vi "Get Tray.vi"(8 "error in":errorcluster, 9 "Grasp":bool=TRUE, 11 "picture":refnum<vi>) -> (0 "error out":errorcluster, 5 "picture":picture)   [LabVIEW 2013]
uses:
  Arm Globals.vi
  ROS/Code/SubVIs/BaxterSide.ctl
  Prim/Fwd Kenimatics - array.vi
  Move/Move Axis.vi
  <vilib>/Analysis/Matrix/NI_Matrix.lvlib
  <vilib>/Analysis/Matrix/Numeric/Multiply/Multiply - RM,RM.vi
  Move/Move XYA.vi
panel:
  out "Range":dbl
  out "result":cluster{"x":dbl, "y":dbl, "a":dbl}
  # "Y"
  # "X"
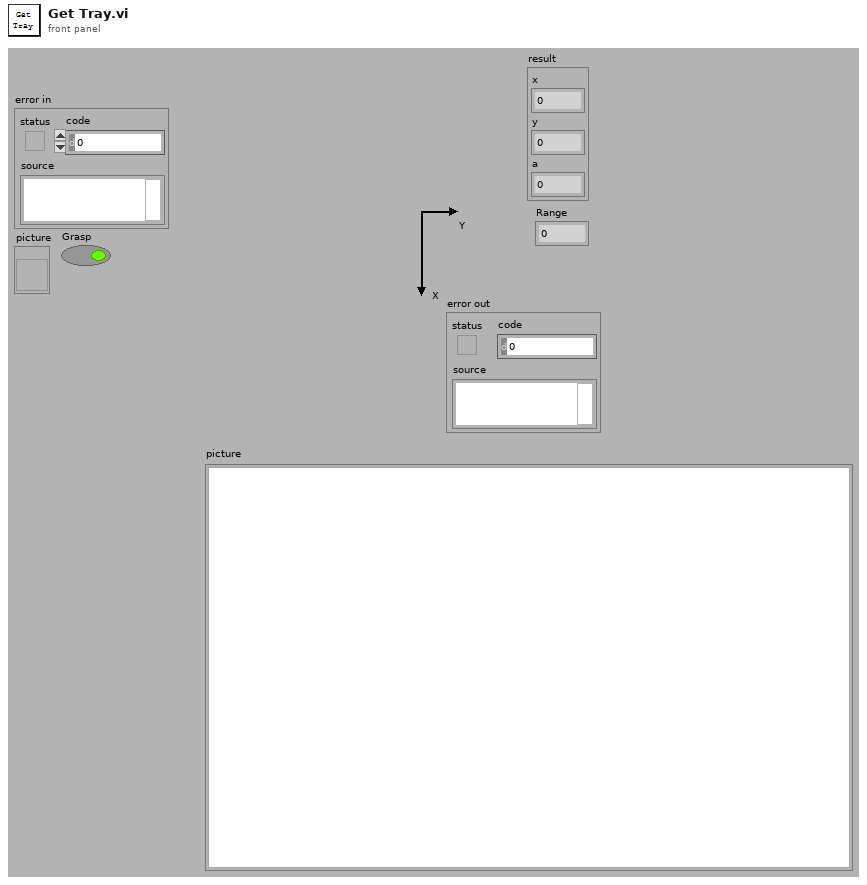
[diagram p1: front panel]
types:
  T1 = typedef "BaxterSide.ctl" = enum16{"left", "right"}
  T2 = typedef "NI_Matrix.lvlib/RealMatrix.ctl" = dbl[][]
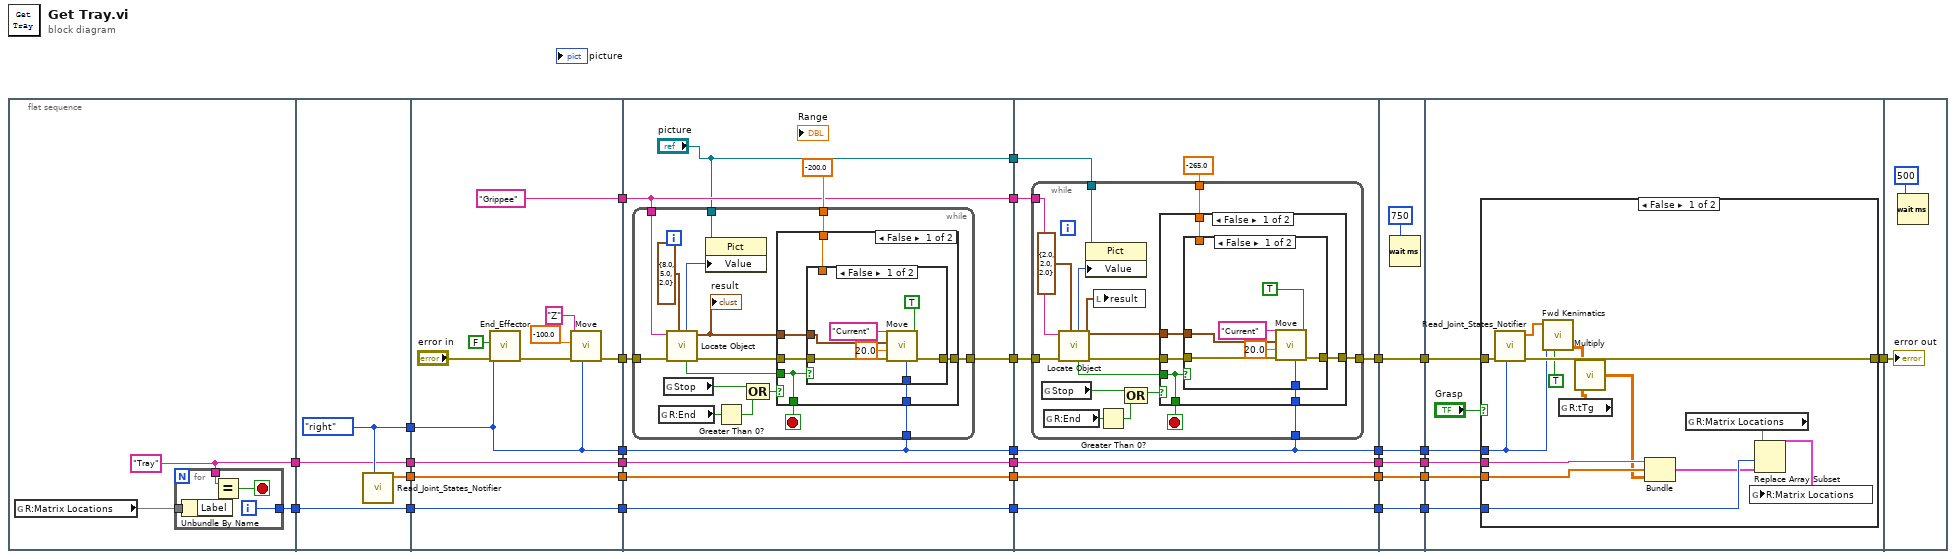
[diagram p0: block diagram]
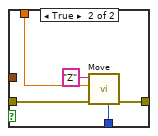
[diagram p2: hidden frame]
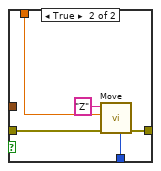
[diagram p4: hidden frame]
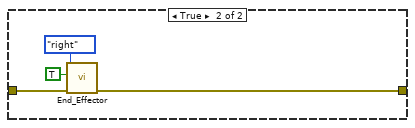
[diagram p6: hidden frame]
diagram:
  n1 = flat-sequence {
    tunnel: [w32] -> w15
    tunnel: [w31] -> w13
    tunnel: [w42] -> w18
    tunnel: [w41] -> w17
    tunnel: [w40] -> w16
    tunnel: w15 -> [w40]
    tunnel: [w39] -> w14
    tunnel: w13 -> [w39]
    tunnel: [w48] -> w30
    tunnel: [w50] -> w29
    tunnel: ["Grippee" ("element")] -> w28
    tunnel: w18 -> [w48]
    tunnel: w17 -> [w46]
    tunnel: w16 -> [w45]
    tunnel: w14 -> [w47]
    tunnel: [w47] -> w12
    tunnel: [w46] -> w11
    tunnel: [w45] -> w10
    tunnel: w30 -> [w59]
    tunnel: w29 -> [w60]
    tunnel: w28 -> [w58]
    tunnel: [w62] -> w27
    tunnel: [w59] -> w26
    tunnel: [w58] -> w25
    tunnel: ["picture"] -> w22
    tunnel: w12 -> [w54]
    tunnel: w11 -> [w55]
    tunnel: w10 -> [w56]
    tunnel: [w56] -> w9
    tunnel: [w55] -> w8
    tunnel: [w54] -> w7
    tunnel: w27 -> [w106]
    tunnel: w26 -> [w102]
    tunnel: w25 -> [w105]
    tunnel: [w104] -> w23
    tunnel: w22 -> [w103]
    tunnel: [w102] -> w20
    tunnel: w9 -> [w101]
    tunnel: w8 -> [w100]
    tunnel: w7 -> [w99]
    tunnel: [w101] -> w5
    tunnel: [w100] -> w3
    tunnel: [w99] -> w1
    tunnel: [w148] -> w24
    tunnel: w23 -> [w148]
    tunnel: [w147] -> w21
    tunnel: w20 -> [w147]
    tunnel: [w146] -> w6
    tunnel: w5 -> [w146]
    tunnel: [w145] -> w4
    tunnel: w3 -> [w145]
    tunnel: [w144] -> w2
    tunnel: w1 -> [w144]
    tunnel: w24 -> [w156]
    tunnel: w21 -> [w154]
    tunnel: [w153] -> w19
    tunnel: w6 -> [w151]
    tunnel: w4 -> [w150]
    tunnel: w2 -> [w152]
    tunnel: w19 -> [w175]
    frame #0 {
      w32 = "Tray"
      n2 = global read "Arm Globals.vi" "R:Matrix Locations"() -> (w33)
      n3 = for {
        tunnel: w33 -> [w35]
        tunnel: w32 -> [w37]
        tunnel: [w34] -> w31
        i -> [w34]
        stop <- w36 stop-if-true
        n4 = Unbundle By Name(w35) -> ("Label"=w38)
        n5 = Equal?(x=w37, y=w38) -> (x = y?=w36:bool)
      }
    }
    frame #1 {
      w42 = BaxterSide."right" ("Side")
      n6 = call "Read_Joint_States_Notifier.vi"("Side"=w42) -> ("Positions"=w41:dbl[])  [unwired: 6 in, 1 out]
    }
    frame #2 {
      n7 = call "End_Effector.vi"("error in"="error in", "Close"=FALSE, "Side"=w48) -> ("error out"=w53:errorcluster)  [unwired: 5 in]
      n8 = call-poly "Move.vi"("Wait Time"=w48, "error in"=w53, "Value"=-100.0 ("Z"), "Location"="Z") -> ("error out"=w50:errorcluster)  [unwired: 7 in]
    }
    frame #3 {
      n9 = while {
        tunnel: w60 -> [w78]
        tunnel: [w76] -> w62
        tunnel: w58 -> [w73]
        tunnel: -200.0 ("Z") -> [w72]
        tunnel: w59 -> [w71]
        tunnel: "picture" -> [w66]
        stop <- w69 stop-if-true
        n10 = global read "Arm Globals.vi" "R:End"() -> (w67:bool)
        n11 = global read "Arm Globals.vi" "Stop"() -> (w74:bool)
        n12 = call "Locate Object.vi"("Tolerance"=cluster{"x":dbl, "y":dbl, "a":dbl} {"x"=8.0, "y"=5.0, "a"=2.0}, "error in"=w78, "Object"=w73) -> ("error out"=w77:errorcluster, "result"=w75:cluster{"x":dbl, "y":dbl, "a":dbl}, "Close"=w68:bool, "picture"=w65:picture)  [unwired: 3 in, 2 out]
        "result" <- w75
        n13 = property class="Pict"(reference=w66, "Value"=w65) -> ()  [unwired: 1 in, 2 out]
        n14 = Greater Than 0?(x=w67) -> (x > 0?=w63:bool)
        n15 = Compound Arithmetic op=OR(w74, w63) -> (w70:bool)
        n16 = case shown="False" w70 {
          selector: w70 -> [_ w97]
          tunnel: w77 -> [w84 w98]
          tunnel: [w83 w98] -> w76
          tunnel: w75 -> [w82 _]
          tunnel: w72 -> [w81 _]
          tunnel: w71 -> [w80 _]
          tunnel: [w79 w97] -> w69
          tunnel: w68 -> [w79 _]
          frame False {
            n17 = case shown="False" w79 {
              tunnel: w84 -> [w91 w96]
              tunnel: [w90 w95] -> w83
              tunnel: w82 -> [w87 _]
              tunnel: w81 -> [_ w94]
              tunnel: w80 -> [w85 w92]
              frame False {
                n18 = call-poly "Move.vi"("Make Vertical"=TRUE, "Side"=w85, "error in"=w91, "Speed (mm/s)"=20.0 ("Speed"), "XYA"=w87, "Location"="Current") -> ("error out"=w90:errorcluster)  [unwired: 5 in]
              }
              frame True {
                n19 = call-poly "Move.vi"("Side"=w92, "error in"=w96, "Value"=w94, "Location"="Z") -> ("error out"=w95:errorcluster)  [unwired: 7 in]
              }
            }
          }
          frame True {
          }
        }
      }
    }
    frame #4 {
      n20 = while {
        tunnel: w106 -> [w123]
        tunnel: [w121] -> w104
        tunnel: w105 -> [w118]
        tunnel: -265.0 ("Z") -> [w117]
        tunnel: w102 -> [w116]
        tunnel: w103 -> [w111]
        stop <- w113 stop-if-true
        n21 = global read "Arm Globals.vi" "Stop"() -> (w119:bool)
        n22 = global read "Arm Globals.vi" "R:End"() -> (w112:bool)
        n23 = call "Locate Object.vi"("Tolerance"=cluster{"x":dbl, "y":dbl, "a":dbl} {"x"=2.0, "y"=2.0, "a"=2.0}, "error in"=w123, "Object"=w118) -> ("error out"=w122:errorcluster, "result"=w120:cluster{"x":dbl, "y":dbl, "a":dbl}, "Close"=w114:bool, "picture"=w110:picture)  [unwired: 3 in, 2 out]
        n24 = property class="Pict"(reference=w111, "Value"=w110) -> ()  [unwired: 1 in, 2 out]
        n25 = local write "result"(w120) -> ()
        n26 = Greater Than 0?(x=w112) -> (x > 0?=w108:bool)
        n27 = Compound Arithmetic op=OR(w119, w108) -> (w115:bool)
        n28 = case shown="False" w115 {
          selector: w115 -> [_ w142]
          tunnel: w114 -> [w124 _]
          tunnel: w122 -> [w129 w143]
          tunnel: [w128 w143] -> w121
          tunnel: w120 -> [w127 _]
          tunnel: w117 -> [w126 _]
          tunnel: w116 -> [w125 _]
          tunnel: [w124 w142] -> w113
          frame False {
            n29 = case shown="False" w124 {
              tunnel: w129 -> [w136 w141]
              tunnel: [w135 w140] -> w128
              tunnel: w127 -> [w132 _]
              tunnel: w126 -> [_ w139]
              tunnel: w125 -> [w130 w137]
              frame False {
                n30 = call-poly "Move.vi"("Make Vertical"=TRUE, "Side"=w130, "error in"=w136, "Speed (mm/s)"=20.0, "XYA"=w132, "Location"="Current") -> ("error out"=w135:errorcluster)  [unwired: 5 in]
              }
              frame True {
                n31 = call-poly "Move.vi"("Side"=w137, "error in"=w141, "Value"=w139, "Location"="Z") -> ("error out"=w140:errorcluster)  [unwired: 7 in]
              }
            }
          }
          frame True {
          }
        }
      }
    }
    frame #5 {
      n32 = Wait (ms)(milliseconds to wait=u32 750) -> ()  [unwired: 1 out]
    }
    frame #6 {
      n33 = case shown="False" "Grasp" {
        tunnel: w156 -> [w168 w172]
        tunnel: [w169 w171] -> w153
        tunnel: w154 -> [w165 _]
        tunnel: w152 -> [w161 _]
        tunnel: w151 -> [w159 _]
        tunnel: w150 -> [w158 _]
        frame False {
          n34 = call "Read_Joint_States_Notifier.vi"("Side"=w165, "error in"=w168) -> ("error out"=w169:errorcluster, "Positions"=w170:dbl[])  [unwired: 5 in]
          n35 = call-poly "Fwd Kenimatics.vi"("Make Vertical"=TRUE, "Side"=w165, "Joints"=w170) -> ("Matrix"=w167:T2)  [unwired: 7 in, 1 out]
          n36 = global read "Arm Globals.vi" "R:tTg"() -> (w166:T2)
          n37 = call-poly <vilib>:"Multiply.vi"("Real Matrix B"=w166, "Real Matrix A"=w167) -> ("A * B"=w157:T2)
          n38 = Bundle(w159, "Positions"=w158, "A * B"=w157) -> (w160:cluster{string, "Positions":dbl[], "A * B":T2})  [unwired: 1 in]
          n39 = global read "Arm Globals.vi" "R:Matrix Locations"() -> (w162)
          n40 = Replace Array Subset(array=w162, new element=w160, index=w161) -> (w163:cluster{string, "Positions":dbl[], "A * B":T2}[])
          n41 = global write "Arm Globals.vi" "R:Matrix Locations"(w163) -> ()
        }
        frame True {
          n42 = call "End_Effector.vi"("error in"=w172, "Close"=TRUE, "Side"=BaxterSide."right") -> ("error out"=w171:errorcluster)  [unwired: 5 in]
        }
      }
    }
    frame #7 {
      n43 = Wait (ms)(milliseconds to wait=u32 500) -> ()  [unwired: 1 out]
      "error out" <- w175
    }
  }
